vi "IsConnected.vi"(8 "error in (no error)":errorcluster, 11 "NetworkStreamWriter in":refnum<class "NetworkStreamWriter.lvclass">) -> (0 "error out":errorcluster, 2 "Connected?":bool, 3 "NetworkStreamWriter out":refnum<class "NetworkStreamWriter.lvclass">)   [LabVIEW 2012, in "NetworkStreamWriter.lvclass"]
doc: "Returns whether or not the NetworkStreamWriter Object is currently connected to a corresponding NetworkStreamReader across the network.\n\nJared Kirschner, 2012."
uses:
  NetworkStreamWriter.lvclass
  NetworkStreamWriter.lvclass/NetworkStreamWriter.ctl
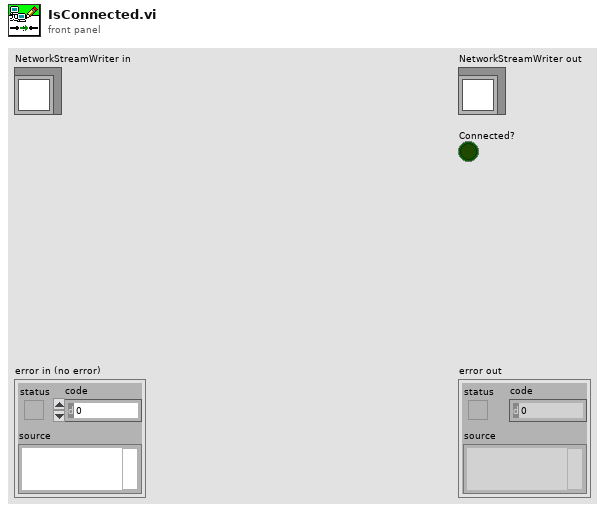
[diagram p1: front panel]
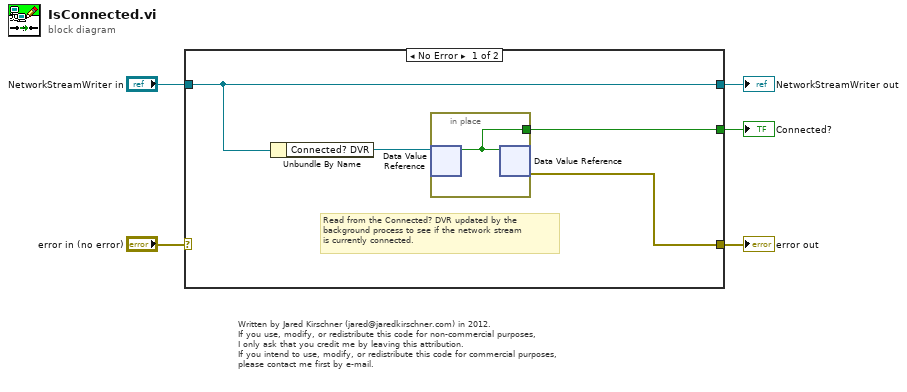
[diagram p0: block diagram]
diagram:
  # "Written by Jared Kirschner (jared@jaredkirschner.com) in 2012.\nIf you use, modify, or redistribute this code for non-commercial purposes,\nI only ask that you credit me by leaving this attribution.\nIf you intend to use, modify, or redistribute this code for commercial purposes,\nplease contact me first by e-mail."
  n1 = case shown="No Error" "error in (no error)" {
    selector: "error in (no error)" -> [_ w12]
    tunnel: [w7 w12] -> w3
    tunnel: [w9 w11] -> w5
    tunnel: "NetworkStreamWriter in" -> [w9 w11]
    tunnel: [w6 _] -> w1
    frame No Error {
      # "Read from the Connected? DVR updated by the\nbackground process to see if the network stream\nis currently connected."
      n2 = Unbundle By Name(w9) -> ("Connected? DVR"=w8:refnum<data-value>)
      n3 = in-place {
        in-place-border: [w10] -> w6
        n4 = in-place-dvr #1(w8) -> (w10:bool)  [unwired: 1 out]
        n5 = in-place-dvr #1(w10) -> (w7:errorcluster)  [unwired: 1 out]
      }
    }
    frame Error {
    }
  }
  "error out" <- w3
  "NetworkStreamWriter out" <- w5
  "Connected?" <- w1
